vi "Hand_Get_Positions_Data.vi"(10 "Motors info in":T1(array[cluster])) -> (2 "Positions (bits)":dbl[](array[numeric]))   [LabVIEW 2015]
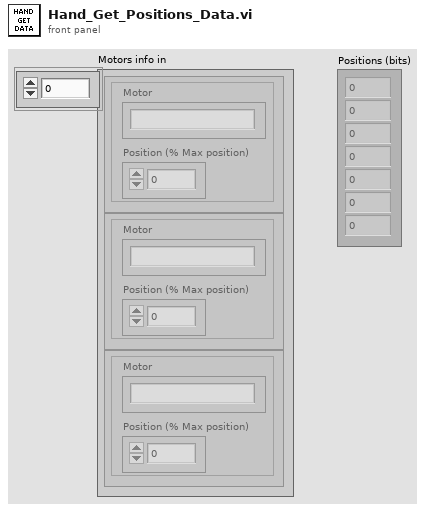
[diagram p1: front panel]
types:
  T1 = cluster{"Motor ":string, "Position (% Max position)":dbl}[]
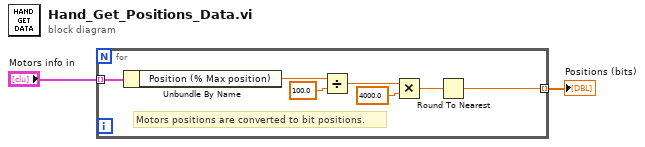
[diagram p0: block diagram]
diagram:
  n1 = for {
    tunnel: "Motors info in" -> [w6] mode=indexing
    tunnel: [w3] -> w1 mode=indexing
    # "Motors positions are converted to bit positions."
    n2 = Unbundle By Name(w6) -> ("Position (% Max position)"=w5:dbl)
    n3 = Divide(x=w5, y=100.0) -> (x/y=w8:dbl)
    n4 = Multiply(x=w8, y=4000.0) -> (x*y=w4:dbl)
    n5 = Round To Nearest(number=w4) -> (nearest integer value=w3:dbl)
  }
  "Positions (bits)" <- w1
